vi "Stepping Array.vi"(8 "Steps":u16, 10 "Range":dbl, 11 "Center":dbl) -> (3 "Array":dbl[](graph))   [LabVIEW 2012]
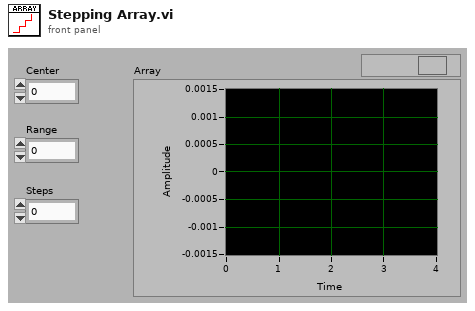
[diagram p1: front panel]
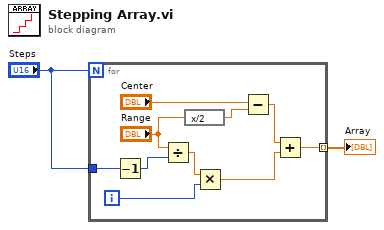
[diagram p0: block diagram]
diagram:
  n1 = for {
    N: "Steps" -> [_]
    tunnel: "Steps" -> [w9]
    tunnel: [w3] -> w1 mode=indexing
    i -> [w6]
    n2 = Decrement(x=w9) -> (x-1=w8:u16)
    n3 = Divide(x="Range", y=w8) -> (x/y=w7:dbl)
    n4 = expression code="x/2"("Range") -> (w12:dbl)
    n5 = Multiply(x=w7, y=w6) -> (x*y=w4:dbl)
    n6 = Subtract(x="Center", y=w12) -> (x-y=w5:dbl)
    n7 = Add(x=w5, y=w4) -> (x+y=w3:dbl)
  }
  "Array" <- w1
